vi "Shift Tag Offsets.vi"(6 "Litt/BigEnd":bool, 8 "error in":errorcluster, 9 "Tags":T1[](array[typedef]), 10 "# of bytes inserted before tag data":i64, 11 "Image Data":u8[](array[numeric])) -> (0 "error out":errorcluster, 3 "Image Data Out":u8[](array[numeric]))   [LabVIEW 2015, in "Tiff reader.lvlib"]
doc: "This .vi replaces the tag \"Offset\" values with a value that has been shifted by the input control. This is useful when stitching together multiple images into a stack, where image # 2 and higher must have their \"Strips Offset\" replaced with the new location of the image data."
uses:
  Tiff reader.lvlib
  FieldTypes.ctl
  IFD Entry.ctl
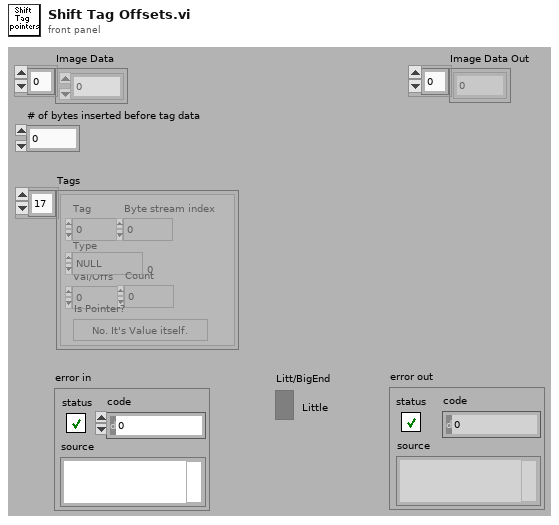
[diagram p1: front panel]
types:
  T1 = typedef "Tiff reader.lvlib/IFD Entry.ctl" = cluster{"Tag":u16, "Type":T2, "Count":u32, "Val/Offs":u32, "Is Pointer?":bool, "Byte stream index":i32}
  T2 = typedef "Tiff reader.lvlib/FieldTypes.ctl" = enum16{"NULL", "U8", "ASCII7", "U16", "U32", "RATIONAL", "SByte(I8)", "Undef(8Bit)", "I16", "I32", "SRat(4B:4B)", "SGL(4Byte)", "DBL(8Byte)"}
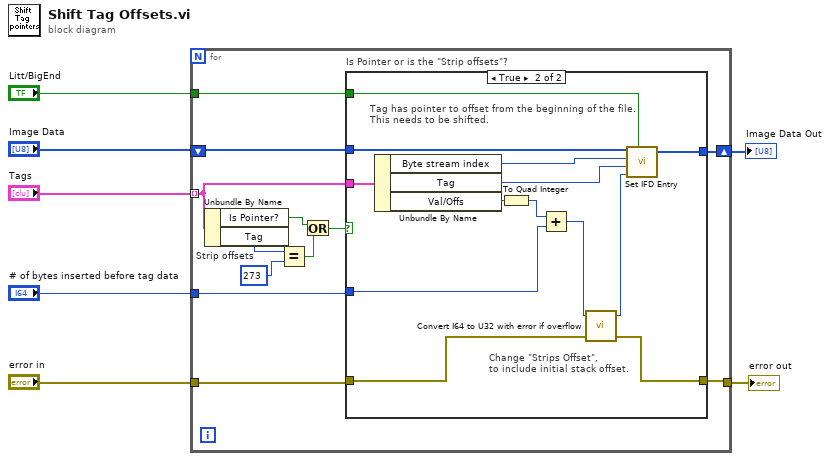
[diagram p0: block diagram]
diagram:
  n1 = for {
    tunnel: "Litt/BigEnd" -> [w19]
    tunnel: "# of bytes inserted before tag data" -> [w17]
    tunnel: "Tags" -> [w13] mode=indexing
    shift-right: [w16] -> w4
    shift-left: "Image Data" -> [w18]
    tunnel: "error in" -> [w15]
    tunnel: [w14] -> w2
    w8 = u16 273  # Strip offsets
    n2 = Unbundle By Name(w13) -> ("Is Pointer?"=w12:bool, "Tag"=w10:u16)
    n3 = Equal?(x=w10, y=w8) -> (x = y?=w9:bool)
    n4 = Or(x=w12, y=w9) -> (x .or. y?=w11:bool)
    n5 = case "Is Pointer or is the \"Strip offsets\"?" shown="True" w11 {
      tunnel: w19 -> [_ w34]
      tunnel: w18 -> [w21 w33]
      tunnel: w17 -> [_ w32]
      tunnel: [w21 w31] -> w16
      tunnel: w15 -> [w20 w30]
      tunnel: [w20 w29] -> w14
      tunnel: w13 -> [_ w22]
      frame False {
        # "Tag has it's value.\nNothing to change."
      }
      frame True {
        # "Tag has pointer to offset from the beginning of the file.\nThis needs to be shifted."
        # "Change \"Strips Offset\",\nto include initial stack offset."
        n6 = Unbundle By Name(w22) -> ("Byte stream index"=w28:i32, "Tag"=w23:u16, "Val/Offs"=w27:u32)
        n7 = To Quad Integer(1:w27) -> (0:w26:i64)
        n8 = Add(x=w26, y=w32) -> (x+y=w25:i64)
        n9 = call "Convert I64 to U32 with error if overflow.vi"("error in"=w30, "I64"=w25) -> ("error out"=w29:errorcluster, "U32"=w24:u32)  [unwired: 2 out]
        n10 = call "Set IFD Entry.vi"("Image Data in"=w33, "Offset in"=w28, "Tag"=w23, "Val / Offset"=w24, "Litt/BigEnd"=w34) -> ("Image Data Out"=w31:u8[])  [unwired: 2 out]
      }
    }
  }
  "Image Data Out" <- w4
  "error out" <- w2
